vi "Rename String Array Property.vi"(8 "error in (no error)":errorcluster, 9 "New Name":string, 10 "Old Name":string, 11 "Item Ref in":T1 format="%.0x") -> (0 "error out":errorcluster, 3 "Item Ref out":T1 format="%.0x")   [LabVIEW 2015, in "Engine Simulation Toolkit System Explorer.lvlib"]
uses:
  Engine Simulation Toolkit System Explorer.lvlib
  <vilib>/NI Veristand/Custom Device API/Custom Device Item Ref.ctl
  <vilib>/NI Veristand/Custom Device API/Get Item Property (String Array).vi
  <vilib>/NI Veristand/Custom Device API/Set Item Property (String Array).vi
  <vilib>/NI VeriStand/Custom Device API/Custom Device API.lvlib
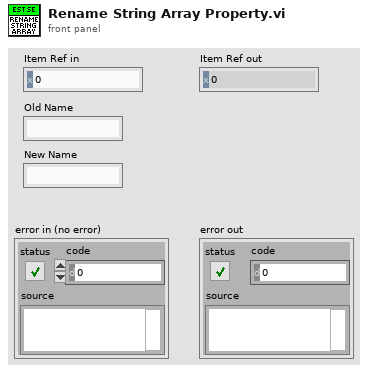
[diagram p1: front panel]
types:
  T1 = typedef "Custom Device API.lvlib/Custom Device Item Ref.ctl" = u64
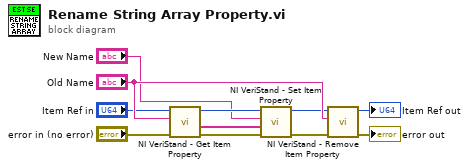
[diagram p0: block diagram]
diagram:
  n1 = call-poly <vilib>:"NI VeriStand - Get Item Property.vi"("error in (no error)"="error in (no error)", "Property Name"="Old Name", "Item Ref in"="Item Ref in") -> ("error out"=w1:errorcluster, "Value"=w2:string[], "Item Ref out"=w6:T1)  [unwired: 5 in, 1 out]
  n2 = call-poly <vilib>:"NI VeriStand - Set Item Property.vi"("error in (no error)"=w1, "Value"=w2, "Property Name"="New Name", "Item Ref in"=w6) -> ("error out"=w4:errorcluster, "Item Ref out"=w5:T1)  [unwired: 5 in, 1 out]
  n3 = call <vilib>:"NI VeriStand - Remove Item Property.vi"("error in (no error)"=w4, "Property Name"="Old Name", "Item Ref in"=w5) -> ("error out"=→"error out":errorcluster, "Item Ref out"=→"Item Ref out":T1)  [unwired: 6 in, 1 out]
